vi "CalibratedMultipleMeasurements.vi"(7 "Show on call?":bool=TRUE, 8 "error in":errorcluster, 9 "Time between calibrations (ms)":u32=1000, 10 "Time / ms (30000)":u32=30000, 11 "VISA resource name":refnum<visa-resource-name>) -> (0 "error out":errorcluster, 1 "Times / LSB":dbl[](array[numeric]), 2 "Times / s":dbl[](array[numeric]), 3 "VISA resource name out":refnum<visa-resource-name>)   [LabVIEW 2017, in "GP22_TDC_Arduinoed.lvlib"]
doc: "Take measurements for the given amount of time, returning an array of doubles and handling calibration automatically."
uses:
  GP22_TDC_Arduinoed.lvlib
  <vilib>/Analysis/NI_AALPro.lvlib
panel:
  out "Histogram Graph":T1(graph)
  out "Calibration / LSB":dbl[](array[numeric])
  out "MMProgress":u8(slide) scale=0.0..100.0
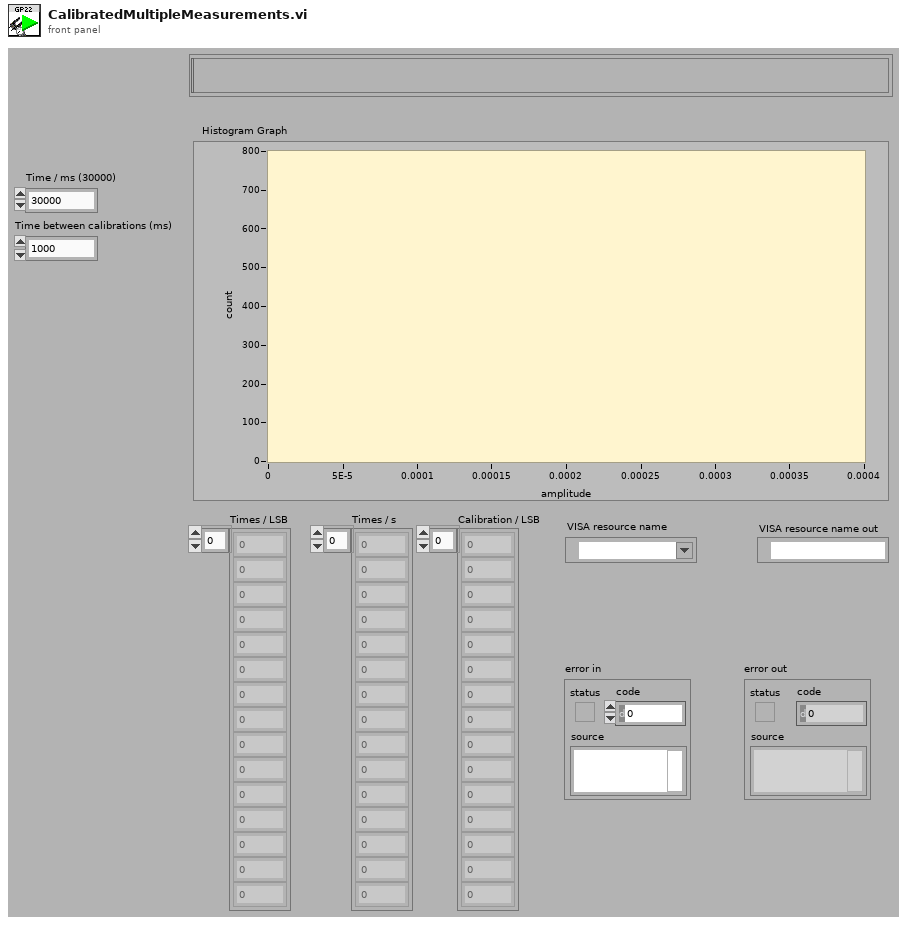
[diagram p1: front panel]
types:
  T1 = cluster{"X Values":dbl[], "Histogram: h(x)":i32[]}
  T2 = enum32{"Invalid", "Standard", "Closed", "Hidden", "Minimized", "Maximized"}
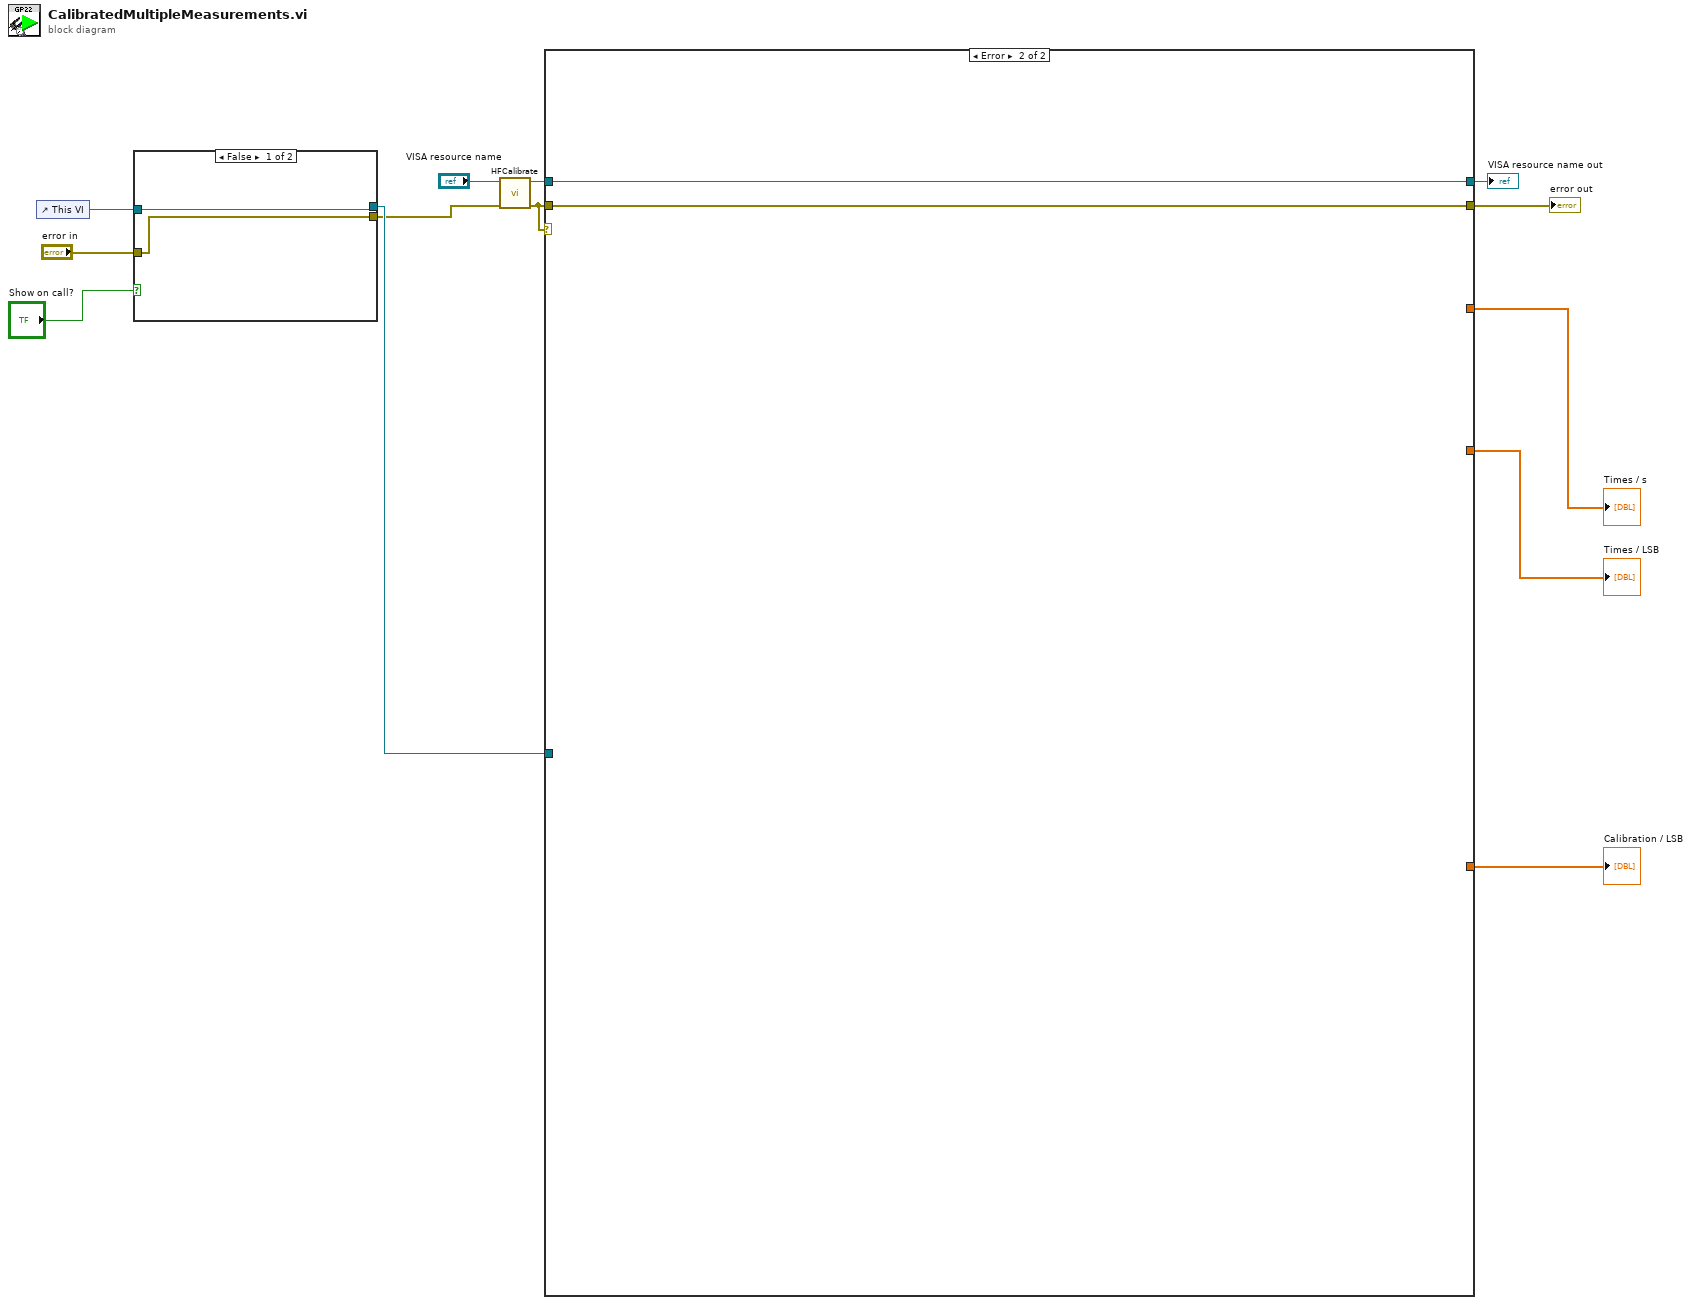
[diagram p0: block diagram]
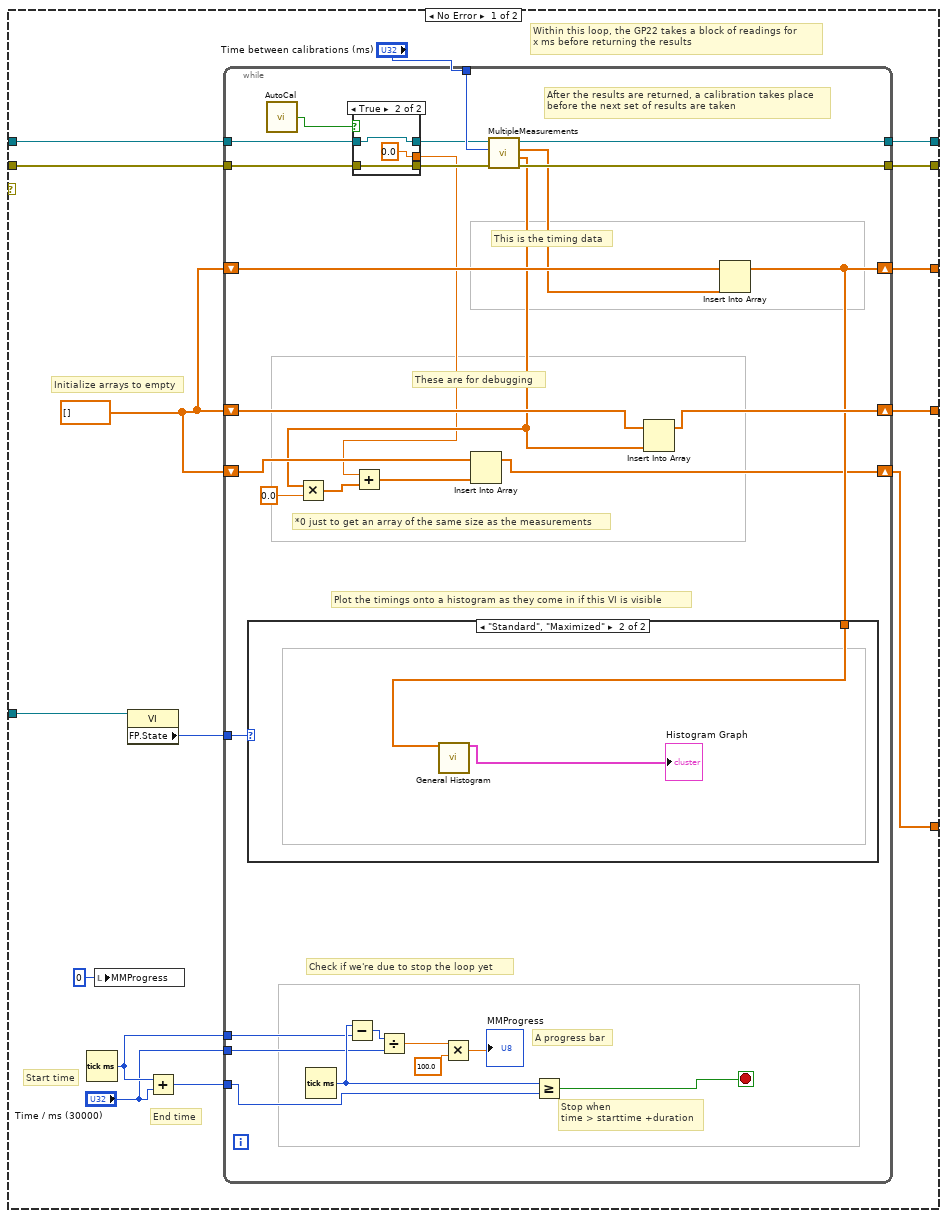
[diagram p2: hidden frame]
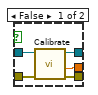
[diagram p4: hidden frame]
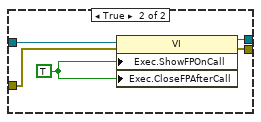
[diagram p5: hidden frame]
diagram:
  n1 = control-ref of="This VI"() -> (w6:refnum<vi>)
  n2 = case shown="False" "Show on call?" {
    tunnel: w6 -> [w14 w20]
    tunnel: [w14 w18] -> w5
    tunnel: "error in" -> [w15 w17]
    tunnel: [w15 w16] -> w3
    frame False {
    }
    frame True {
      w19 = TRUE ("Execution:Close After Call")
      n3 = property class="VI"(reference=w20, error in=w17, "Exec.ShowFPOnCall"=w19, "Exec.CloseFPAfterCall"=w19) -> (reference out=w18:refnum<vi>, error out=w16:errorcluster)
    }
  }
  n4 = call "HFCalibrate.vi"("error in (no error)"=w3, "VISA resource name"="VISA resource name") -> ("error out"=w1:errorcluster, "VISA resource name out"=w8:refnum<visa-resource-name>)  [unwired: 5 in, 2 out]
  n5 = case shown="Error" w1 {
    tunnel: [w31 w77] -> w13
    tunnel: [w30 w76] -> w12
    tunnel: [w29 _] -> w11
    tunnel: [w28 _] -> w10
    tunnel: [w27 _] -> w9
    tunnel: w1 -> [w24 w76]
    tunnel: w8 -> [w23 w77]
    tunnel: w5 -> [w21 _]
    frame No Error {
      w26 = dbl[] []
      # "Initialize arrays to empty"
      # "Within this loop, the GP22 takes a block of readings for\nx ms before returning the results"
      # "End time"
      # "Start time"
      n6 = Tick Count (ms)() -> (millisecond timer value=w33:u32)
      n7 = local write "MMProgress"(u8 0 ("MMProgress")) -> ()
      n8 = property class="VI"(reference=w21) -> ("FP.State"=w25:T2)  [unwired: 1 in, 2 out]
      n9 = Add(x=w33, y="Time / ms (30000)") -> (x+y=w35:u32)
      n10 = while {
        tunnel: [w65] -> w31
        tunnel: "Time between calibrations (ms)" -> [w64]
        tunnel: w24 -> [w61]
        tunnel: [w63] -> w30
        tunnel: w35 -> [w48]
        shift-right: [w47] -> w29
        shift-left: w26 -> [w58]
        shift-right: [w55] -> w28
        shift-left: w26 -> [w56]
        shift-right: [w39] -> w27
        shift-left: w26 -> [w54]
        tunnel: w33 -> [w45]
        tunnel: "Time / ms (30000)" -> [w43]
        tunnel: w25 -> [w38]
        tunnel: w23 -> [w37]
        stop <- w62 stop-if-true
        # "Plot the timings onto a histogram as they come in if this VI is visible"
        # "Check if we're due to stop the loop yet"
        # "A progress bar"
        # "These are for debugging"
        # "This is the timing data"
        # "After the results are returned, a calibration takes place\nbefore the next set of results are taken"
        # "*0 just to get an array of the same size as the measurements"
        # "Stop when \ntime > starttime +duration"
        n11 = call "AutoCal.vi"() -> ("Autocal mode?"=w36:bool)  [unwired: 2 in]
        n12 = Tick Count (ms)() -> (millisecond timer value=w46:u32)
        n13 = Subtract(x=w46, y=w45) -> (x-y=w44:u32)
        n14 = case shown="True" w36 {
          tunnel: w61 -> [w72 w75]
          tunnel: [w71 w75] -> w60
          tunnel: [w70 w73] -> w59
          tunnel: [w69 0.0 ("y")] -> w50
          tunnel: w37 -> [w68 w73]
          frame False {
            n15 = call "Calibrate.vi"("error in (no error)"=w72, "VISA resource name"=w68) -> ("error out"=w71:errorcluster, "output raw"=w69:dbl, "VISA resource name out"=w70:refnum<visa-resource-name>)  [unwired: 5 in, 1 out]
          }
          frame True {
          }
        }
        n16 = Divide(x=w44, y=w43) -> (x/y=w42:dbl)
        n17 = Multiply(x=w42, y=100.0) -> (x*y=→"MMProgress":dbl)
        n18 = call "MultipleMeasurements.vi"("error in (no error)"=w60, "Time in ms (30000)"=w64, "VISA resource name"=w59) -> ("error out"=w63:errorcluster, "Raw output"=w53:dbl[], "output/s"=w57:dbl[], "VISA resource name out"=w65:refnum<visa-resource-name>)  [unwired: 5 in]
        n19 = Multiply(x=w53, y=0.0) -> (x*y=w51:dbl[])
        n20 = Add(x=w50, y=w51) -> (x+y=w49:dbl[])
        n21 = Insert Into Array(array=w54, new element=w49) -> (w39:dbl[])  [unwired: 1 in]
        n22 = Greater Or Equal?(x=w46, y=w48) -> (x >= y?=w62:bool)
        n23 = Insert Into Array(array=w56, new element=w53) -> (w55:dbl[])  [unwired: 1 in]
        n24 = Insert Into Array(array=w58, new element=w57) -> (w47:dbl[])  [unwired: 1 in]
        n25 = case shown="\"Standard\", \"Maximized\"" w38 {
          tunnel: w47 -> [_ w67]
          frame "Invalid", Default {
            # "Do nothing here if this VI isn't visible"
          }
          frame "Standard", "Maximized" {
            n26 = call <vilib>:"General Histogram.vi"("X"=w67) -> ("Histogram Graph"=→"Histogram Graph":T1)  [unwired: 10 in, 4 out]
          }
        }
      }
    }
    frame Error {
    }
  }
  "VISA resource name out" <- w13
  "error out" <- w12
  "Times / s" <- w11
  "Times / LSB" <- w10
  "Calibration / LSB" <- w9
